vi "Close.vi.REMOTE.vi"(8 "error in (no error)":errorcluster, 11 "Masterflex Settings in":T1) -> (0 "error out":errorcluster, 3 "Masterflex Settings out":T1)   [LabVIEW 2018, in "Masterflex 7550-30.lvlib"]
uses:
  Masterflex 7550-30.lvlib
  Controls/Settings Cluster.ctl
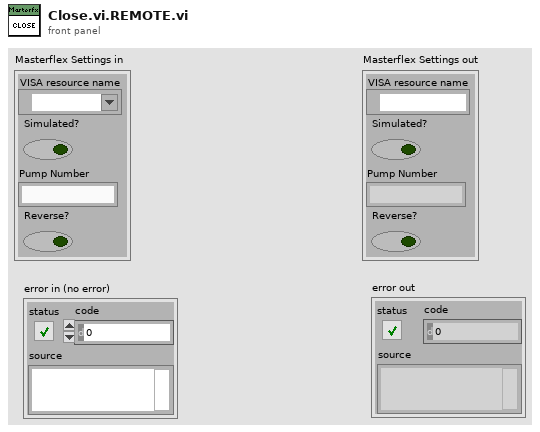
[diagram p1: front panel]
types:
  T1 = typedef "Masterflex 7550-30.lvlib/Settings Cluster.ctl" = cluster{"VISA resource name":refnum<visa-resource-name>, "Simulated?":bool, "Pump Number":string, "Reverse?":bool}
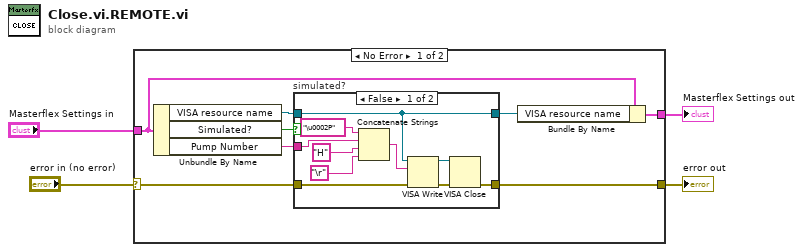
[diagram p0: block diagram]
diagram:
  n1 = case shown="No Error" "error in (no error)" {
    selector: "error in (no error)" -> [w11 w26]
    tunnel: [w10 w26] -> w4
    tunnel: [w9 w25] -> w1
    tunnel: "Masterflex Settings in" -> [w8 w25]
    frame No Error {
      n2 = Unbundle By Name(w8) -> ("VISA resource name"=w6:refnum<visa-resource-name>, "Simulated?"=w12:bool, "Pump Number"=w5:string)
      n3 = case "simulated?" shown="False" w12 {
        tunnel: [w22 w24] -> w10
        tunnel: w11 -> [w15 w24]
        tunnel: [w18 w23] -> w7
        tunnel: w6 -> [w18 w23]
        tunnel: w5 -> [w14 _]
        frame False {
          n4 = Concatenate Strings("\u0002P" ("string"), w14, "H" ("string"), "\r") -> (w13:string)
          n5 = VISA Write(VISA resource name=w18, write buffer=w13, error in (no error)=w15) -> (VISA resource name out=w17:refnum<visa-resource-name>, error out=w16:errorcluster)  [unwired: 1 out]
          n6 = VISA Close(VISA resource name=w17, error in (no error)=w16) -> (error out=w22:errorcluster)
        }
        frame True {
        }
      }
      n7 = Bundle By Name(cluster=w8, "VISA resource name"=w7) -> (w9:T1)
    }
    frame Error {
    }
  }
  "error out" <- w4
  "Masterflex Settings out" <- w1
